vi "Chart.vi"(10 "Array":dbl[](array[numeric])) -> (3 "Waveform Chart":dbl(graph))   [LabVIEW 2012]
panel:
  in  "Y  min":dbl=-5.0
  in  "Y max":dbl=5.0
  out "Number of points":dbl
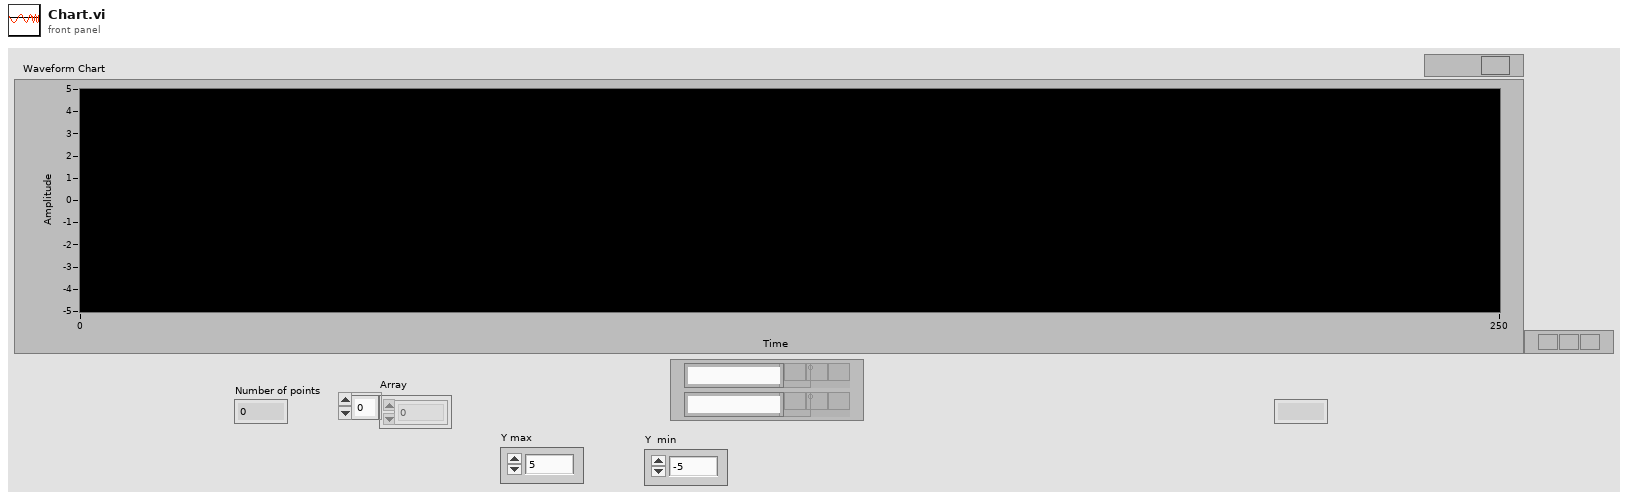
[diagram p1: front panel]
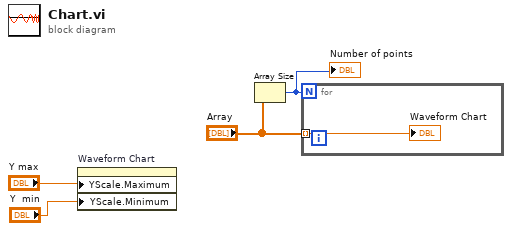
[diagram p0: block diagram]
diagram:
  n1 = property on="Waveform Chart" class="WFChart (strict)"("YScale.Maximum"="Y max", "YScale.Minimum"="Y  min") -> ()  [unwired: 2 in, 2 out]
  n2 = Array Size(array="Array") -> (size(s)=w3:i32)
  "Number of points" <- w3
  n3 = for {
    N: w3 -> [_]
    tunnel: "Array" -> [w5] mode=indexing
    "Waveform Chart" <- w5
  }
